vi "test_Loopback(Tx Generic - Rx Mon).vi"() -> ()   [LabVIEW 2020]
doc: "Overview: This examples helps to setup the board (or boards) and validate that it can send and receive parameters.\n\nRequirement: One AIM ARINC-664 board with installed AIM ARINC 664 BSP.\nRestrictions: None.\nInstruction:\n1. Select the Board ID (0 if you have only one board in your system) and the port number. If you want to validate between two ports in one device, you can use tx board and Rx Boardd\n2. Run the VI.\n3. See the result in the indicators.\nFor detailed information about functions use, see documents in <BSP Installation folder>\\AIM GmbH\\Arinc 664 Windows BSP <version>\\Doc."
uses:
  <instrlib>/AIM GmbH/_AIM 664/_controls/session_monitor_config.ctl
  <instrlib>/AIM GmbH/_AIM 664/_controls/queue_header_generic.ctl
  <instrlib>/AIM GmbH/_AIM 664/_controls/queue_data_full.ctl
  <instrlib>/AIM GmbH/_AIM 664/_controls/port_speed.ctl
  <instrlib>/AIM GmbH/_AIM 664/bsp/Fdx Create Session (RX-Monitor).vi
  <instrlib>/AIM GmbH/_AIM 664/bsp/Fdx Create Session (Tx-Generic).vi
  <instrlib>/AIM GmbH/_AIM 664/bsp/Fdx Start (Rx).vi
  <instrlib>/AIM GmbH/_AIM 664/bsp/Fdx Start (Tx).vi
  <instrlib>/AIM GmbH/_AIM 664/bsp/Fdx Stop (Tx).vi
  <instrlib>/AIM GmbH/_AIM 664/bsp/Fdx Stop (Rx).vi
  <instrlib>/AIM GmbH/_AIM 664/AIM664LV.lvlib
panel:
  in  "UDPsrcPort":u16=1
  in  "UDPdstPort":u16=1
  in  "Fdx configuration":T1={"domainID"=1, "sideID"=1, "locationID"=1, "interfaceID"=1, "partitionID"=1} {"interfaceID" format="%.0b"}
  in  "VL Id":u16=60
  out "EntryRead":u32
  out "BytesRead":u32
  out "Synchronized":u32
  out "ReadBuffer":u8[](array[numeric]) format="%.0x"
  out "Statistics":string[][](table)
  in  "MaxReadBytes":u32=257
  out "current time":timestamp
  out "tx timed out":bool
  out "rx timed out":bool
  in  "Data Payload":u8[](array[numeric])=[65, 66, 67, 68, 69, 70, 71, 72, 73, 74, 75, 76, 77, 78, 79, 80, 81] format="%.0x"
  in  "HeaderInfo":T2={"InterFrameGap"=1000, "PacketGroupWaitTime"=10000, "PayloadBufferMode"=0, "PayloadGenerationMode"=0, "PreambleCount"=0, "Skew"=1, "NetSelect"=0, "FrameStartMode"=1, "PhysErrorInjection"=0, "SequenceNumberInit"=65535, "SequenceNumberOffset"=65535} {"NetSelect" items=["FDX_TX_FRAME_DLY_A"=0, "FDX_TX_FRAME_DLY_B"=1, "FDX_TX_FRAME_BOTH "=3, "FDX_TX_FRAME_ONLY_A"=4, "FDX_TX_FRAME_ONLY_B "=5]; "FrameStartMode" items=["FDX_TX_FRAME_START_IFG", "FDX_TX_FRAME_START_PGWT", "FDX_TX_FRAME_START_TRG"]; "PhysErrorInjection" items=["FDX_TX_FRAME_ERR_OFF"=0, "FDX_TX_FRAME_ERR_CRC"=1, "FDX_TX_FRAME_ERR_ALI"=2, "FDX_TX_FRAME_ERR_PRE"=4, "FDX_TX_FRAME_ERR_PHY"=8]; "SequenceNumberInit" items=["FDX_TX_FRAME_SEQ_INIT_AUTO"=65535]; "SequenceNumberOffset" items=["FDX_TX_FRAME_SEQ_OFFS_AUTO "=65535]; "PayloadGenerationMode" items=["FDX_TX_FRAME_PGM_USER"=0, "FDX_TX_FRAME_PGM_IP_PART"=1, "FDX_TX_FRAME_PGM_IP_FULL"=2, "FDX_TX_FRAME_PGM_IP_PART_TT"=10, "FDX_TX_FRAME_PGM_IP_FULL_TT"=20]; "PayloadBufferMode" items=["FDX_TX_FRAME_PBM_STD", "FDX_TX_FRAME_PBM_MAC", "FDX_TX_FRAME_PBM_UDP"]}
  out "error out":errorcluster
  in  "EntryCount (1)":u32=1
  out "MonStatus":T3 {"MonStatus" items=["FDX_MON_OFF", "FDX_MON_WAIT_FOR_TRIGGER", "FDX_MON_TRIGGERED", "FDX_MON_STOPPED", "FDX_MON_FULL", "FDX_MON_OVERLOAD"]}
  in  "Control":u32(ring)=1 items=["FDX_RX_GS_RES_NO_CNT", "FDX_RX_GS_RES_ALL_CNT", "FDX_RX_GS_RES_ERR_CNT"]
  out "TxStatus":T4 {"TransmitMode" items=["FDX_TX_GENERIC", "FDX_TX_REPLAY", "FDX_TX_INDIVIDUAL"]; "TxStatus" items=["FDX_STAT_STOP", "FDX_STAT_RUN", "FDX_STAT_ERROR", "FDX_STAT_WAIT_F_TRIG"]}
  out "rx link ok":bool
  out "tx link ok":bool
  out "GlobMonSize":u32
  in  "RecordingFileName":path
  in  "MaxFileSize MB (1)":u32=1
  in  "Strobe":u32(ring) items=["FDX_MON_STROBE_DIS", "FDX_MON_STROBE_STOP", "FDX_MON_STROBE_START"]
  in  "CaptureMode":u32(ring) items=["FDX_MON_SINGLE ", "FDX_MON_CONTINUOUS", "FDX_MON_SELECTIVE", "FDX_MON_RECORDING", "FDX_MON_REROS", "FDX_MON_HMU"]
  in  "TriggerPosition":u32
  in  "MonitorConfig":T5={"DefaultCronoMode"=1, "GlbMonBufferSizeIn"=0} {"DefaultCronoMode" items=["FDX_RX_DEFAULT_ENA_CNT", "FDX_RX_DEFAULT_MON_ENA_ALL", "FDX_RX_DEFAULT_MON_ENA_GOOD"]}
  in  "Rx Port":u32=1
  in  "Rx Board":u32
  out "PortInitOut":T6 {"PortConfig" items=["FDX_SINGLE", "FDX_REDUNDANT"]}
  out "TxQueueInfo":cluster{"QueueBaseAddr":u32, "QueueSizeOut":u32}
  in  "Tx Board":u32
  in  "QueueSizeIn":u32
  in  "Tx Port":u32
  # "ARINC 664 Loopback"
  # "Overview: This examples helps to setup the board (or boards) and validate that it can send and receive parameters.\n\nRequirement: One AIM ARINC-664 board with installed AIM ARINC 664 BSP.\nRestrictions: None.\nInstruction:\n1. Select the Board ID (0 if you have only one board in your system) and the port number. If you want to validate between two ports in one device, you can use tx board and Rx Boardd\n2. Run the VI.\n3. See the result in the indicators."
  # "TX Status"
  # "Monitor Results"
  # "HW config"
  # "TX Configuration"
  # "Monitor Configuration"
  # "Monitor Status"
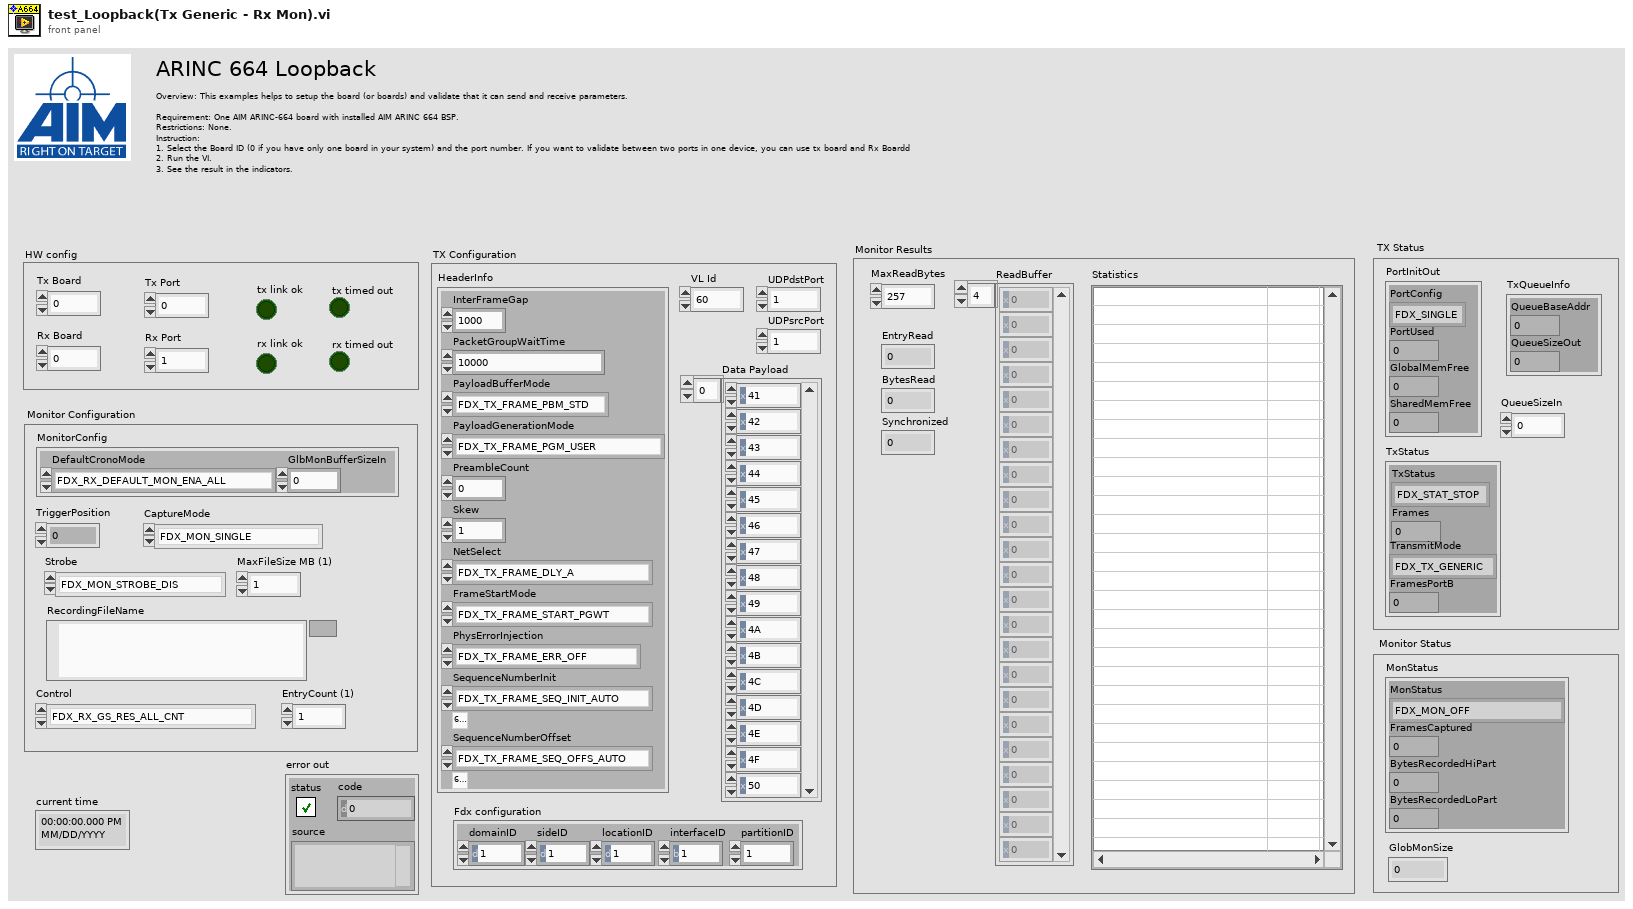
[diagram p1: front panel]
types:
  T1 = typedef "AIM664LV.lvlib/queue_data_full.ctl" = cluster{"domainID":u8, "sideID":u8, "locationID":u8, "interfaceID":u8, "partitionID":u8}
  T2 = typedef "AIM664LV.lvlib/queue_header_generic.ctl" = cluster{"InterFrameGap":u32, "PacketGroupWaitTime":u32, "PayloadBufferMode":u8, "PayloadGenerationMode":u8, "PreambleCount":u8, "Skew":u32, "NetSelect":u8, "FrameStartMode":u8, "PhysErrorInjection":u32, "SequenceNumberInit":u16, "SequenceNumberOffset":u16}
  T3 = cluster{"MonStatus":u32, "FramesCaptured":u32, "BytesRecordedHiPart":u32, "BytesRecordedLoPart":u32}
  T4 = cluster{"TxStatus":u32, "Frames":u32, "TransmitMode":u32, "FramesPortB":u32}
  T5 = typedef "AIM664LV.lvlib/session_monitor_config.ctl" = cluster{"DefaultCronoMode":u32, "GlbMonBufferSizeIn":u32}
  T6 = cluster{"PortConfig":u32, "PortUsed":u32, "GlobalMemFree":u32, "SharedMemFree":u32}
  T7 = typedef "AIM664LV.lvlib/port_speed.ctl" = u32
  T8 = cluster{"PortSpeed[0]":T7, "PortSpeed[1]":T7, "PortSpeed[2]":T7, "PortSpeed[3]":T7}
  T9 = cluster{"TotalByteCount":u32[], "FrameGoodCount":u32[], "FrameErrorCount":u32[], "BytesPerSecond":u32[], "FramesPerSecond":u32[], "PhysErrorCount":u32[], "PreamErrorCount":u32[], "UnaligErrorCount":u32[], "CRCErrorCount":u32[], "IFGErrorCount":u32[], "IPErrorCount":u32[], "MACErrorCount":u32[], "NoSfdErrorCount":u32[], "VLLenErrorCount":u32[], "SNIntegrityErrorCount":u32[], "TrafShapingViolationCount":u32[], "MAC1Short":u32[], "MAC64To127Count":u32[], "MAC128To255Count":u32[], "MAC256To511Count":u32[], "MAC512To1023Count":u32[], "MAC1024To1518Count":u32[], "MACLong":u32[]}
  T10 = cluster{"EntryRead":u32, "BytesRead":u32, "Synchronized":u32, "ReadBuffer":u8[]}
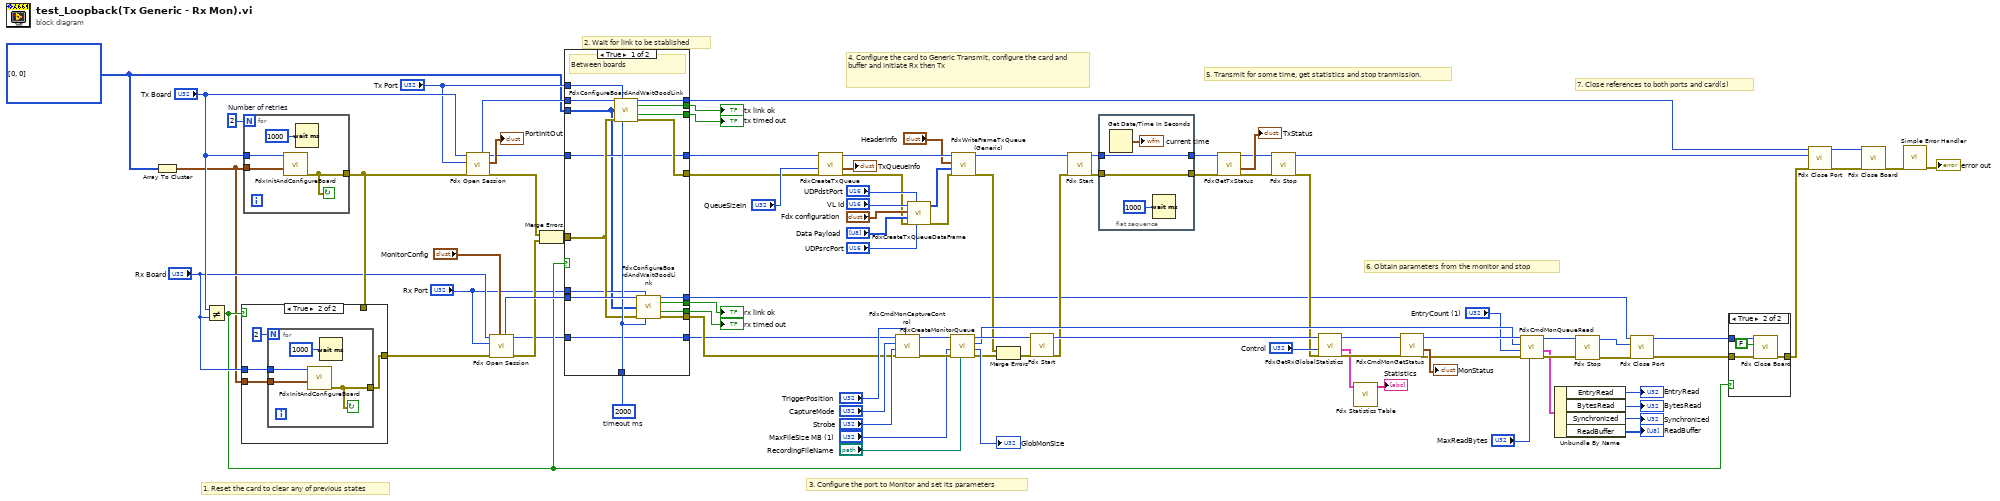
[diagram p0: block diagram]
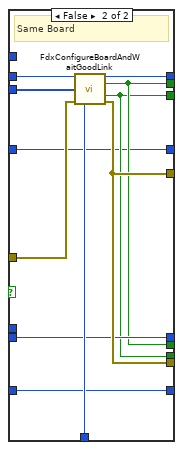
[diagram p3: hidden frame]
diagram:
  w4 = T7[] [0, 0] items=["FDX_100MBIT"=0, "FDX_10MBIT"=1, "FDX_1000MBIT"=5, "FDX_AUTO_100MBIT"=2, "FDX_AUTO_10MBIT"=3] ("PortSpeed")
  w34 = 2  # Number of retries
  w23 = u32 2000  # timeout ms
  # "7. Close references to both ports and card(s)"
  # "6. Obtain parameters from the monitor and stop"
  # "5. Transmit for some time, get statistics and stop tranmission."
  # "2. Wait for link to be stablished"
  # "3. Configure the port to Monitor and set its parameters"
  # "4. Configure the card to Generic Transmit, configure the card and buffer and initiate Rx then Tx"
  # "1. Reset the card to clear any of previous states"
  n1 = Array To Cluster(array=w4) -> (cluster=w3:T8)
  n2 = Not Equal?(x="Tx Board", y="Rx Board") -> (x != y?=w12:bool)
  n3 = for {
    N: w34 -> [_]
    tunnel: [w96] -> w32
    tunnel: "Tx Board" -> [w95]
    tunnel: w3 -> [w94]
    stop <- w96 continue-if-true
    n4 = call <instrlib>:"FdxInitAndConfigureBoard.vi"("PortSpeed (100Mbit)"=w94, "board index"=w95) -> ("error out"=w96:errorcluster)  [unwired: 5 in, 4 out]
    n5 = Wait (ms)(milliseconds to wait=u32 1000) -> ()  [unwired: 1 out]
  }
  n6 = case shown="True" w12 {
    tunnel: w32 -> [w98 _]
    tunnel: [w98 w100] -> w31
    tunnel: "Rx Board" -> [_ w101]
    tunnel: w3 -> [_ w99]
    frame False {
    }
    frame True {
      n7 = for {
        N: 2 -> [_]
        tunnel: [w105] -> w100
        tunnel: w101 -> [w104]
        tunnel: w99 -> [w103]
        stop <- w105 continue-if-true
        n8 = call <instrlib>:"FdxInitAndConfigureBoard.vi"("PortSpeed (100Mbit)"=w103, "board index"=w104) -> ("error out"=w105:errorcluster)  [unwired: 5 in, 4 out]
        n9 = Wait (ms)(milliseconds to wait=u32 1000) -> ()  [unwired: 1 out]
      }
    }
  }
  n10 = call-poly <instrlib>:"Fdx Open Session.vi"("error in (no error)"=w32, "port"="Tx Port", "board"="Tx Board") -> ("error out"=w22:errorcluster, "PortInitOut"=→"PortInitOut":T6, "port handle out"=w11:u32, "InstrumentHandle_board out"=w93:u32)  [unwired: 3 in, 2 out]
  n11 = call-poly <instrlib>:"Fdx Open Session.vi"("MonitorConfig"="MonitorConfig", "error in (no error)"=w31, "port"="Rx Port", "board"="Rx Board") -> ("error out"=w19:errorcluster, "InstrumentHandle_port out"=w9:u32, "InstrumentHandle_board out"=w80:u32)  [unwired: 2 in, 3 out]
  n12 = Merge Errors(w22, w19) -> (w18:errorcluster)
  n13 = case shown="True" w12 {
    tunnel: w93 -> [w123 w134]
    tunnel: w80 -> [w122 w129]
    tunnel: [w121 w128] -> w79
    tunnel: [w120 w133] -> w57
    tunnel: [w119 w129] -> w13
    tunnel: [w118 w127] -> w53
    tunnel: w23 -> [w117 w132]
    tunnel: [w116 w130] -> w21
    tunnel: [w115 w130] -> w20
    tunnel: w18 -> [w114 w131]
    tunnel: [w113 w128] -> w17
    tunnel: [w112 w127] -> w16
    tunnel: w11 -> [w111 w126]
    tunnel: [w111 w126] -> w10
    tunnel: w9 -> [w110 w125]
    tunnel: [w110 w125] -> w8
    tunnel: "Tx Port" -> [w109 _]
    tunnel: "Rx Port" -> [w108 _]
    tunnel: w4 -> [w107 w124]
    frame True {
      # "Between boards"
      n14 = call <instrlib>:"FdxConfigureBoardAndWaitGoodLink.vi"("InstrumentHandle_board in"=w123, "Port for Goodlink (-1 is all)"=w109, "PortSpeed"=w107, "error in"=w114, "timeout (ms)"=w117) -> ("InstrumentHandle_board out"=w120:u32, "good link"=w113:bool, "timed out"=w112:bool, "error out"=w116:errorcluster)  [unwired: 7 in]
      n15 = call <instrlib>:"FdxConfigureBoardAndWaitGoodLink.vi"("InstrumentHandle_board in"=w122, "Port for Goodlink (-1 is all)"=w108, "PortSpeed"=w107, "error in"=w114, "timeout (ms)"=w117) -> ("InstrumentHandle_board out"=w119:u32, "good link"=w121:bool, "timed out"=w118:bool, "error out"=w115:errorcluster)  [unwired: 7 in]
    }
    frame False {
      # "Same Board"
      n16 = call <instrlib>:"FdxConfigureBoardAndWaitGoodLink.vi"("InstrumentHandle_board in"=w134, "PortSpeed"=w124, "error in"=w131, "timeout (ms)"=w132) -> ("InstrumentHandle_board out"=w133:u32, "good link"=w128:bool, "timed out"=w127:bool, "error out"=w130:errorcluster)  [unwired: 8 in]
    }
  }
  "tx link ok" <- w17
  "rx link ok" <- w79
  "rx timed out" <- w53
  "tx timed out" <- w16
  n17 = call <instrlib>:"FdxCreateTxQueue.vi"("error in"=w21, "QueueSizeIn"="QueueSizeIn", "InstrumentHandle_port"=w10) -> ("error out"=w29:errorcluster, "TxQueueInfo"=→"TxQueueInfo":cluster{"QueueBaseAddr":u32, "QueueSizeOut":u32}, "InstrumentHandle_port"=w56:u32)  [unwired: 6 in]
  n18 = call <instrlib>:"FdxCmdMonCaptureControl.vi"("TriggerPosition"="TriggerPosition", "error in"=w20, "Strobe"="Strobe", "CaptureMode"="CaptureMode", "InstrumentHandle_port in"=w8) -> ("error out"=w84:errorcluster, "InstrumentHandle_port out"=w85:u32)  [unwired: 5 in]
  n19 = call <instrlib>:"FdxCreateTxQueueDataFrame.vi"("UDPsrcPort"="UDPsrcPort", "UDPdstPort"="UDPdstPort", "error in"=w29, "Payload"="Data Payload", "afdx configuration"="Fdx configuration", "VL Id"="VL Id") -> ("error out"=w28:errorcluster, "Frame"=w40:u8[])  [unwired: 3 in, 1 out]
  n20 = call <instrlib>:"FdxCreateMonitorQueue.vi"("RecordingFileName"="RecordingFileName", "error in (no error)"=w84, "MaxFileSize MB (1)"="MaxFileSize MB (1)", "InstrumentHandle_port in"=w85) -> ("error out"=w26:errorcluster, "GlobMonSize"=→"GlobMonSize":u32, "QueueIdOut"=w64:u32, "InstrumentHandle_port out"=w78:u32)  [unwired: 4 in]
  n21 = call <instrlib>:"FdxWriteFrameTxQueue (Generic).vi"("error in (no error)"=w28, "Frame in"=w40, "HeaderInfo"="HeaderInfo", "InstrumentHandle_port in"=w56) -> ("error out"=w24:errorcluster, "InstrumentHandle_port out"=w55:u32)  [unwired: 6 in]
  n22 = Merge Errors(w24, w26) -> (w25:errorcluster)
  n23 = call-poly <instrlib>:"Fdx Start.vi"("error in"=w25, "InstrumentHandle_port in"=w78) -> ("error out"=w51:errorcluster, "InstrumentHandle_port out"=w71:u32)  [unwired: 8 in]
  n24 = call-poly <instrlib>:"Fdx Start.vi"("error in"=w51, "InstrumentHandle_port in"=w55) -> ("error out"=w52:errorcluster, "InstrumentHandle_port out"=w77:u32)  [unwired: 8 in]
  n25 = flat-sequence {
    tunnel: w52 -> [w137]
    tunnel: [w137] -> w74
    tunnel: [w136] -> w75
    tunnel: w77 -> [w136]
    frame #0 {
      n26 = Get Date/Time In Seconds() -> (seconds since 1Jan1904=→"current time":timestamp)
      n27 = Wait (ms)(milliseconds to wait=u32 1000) -> ()  [unwired: 1 out]
    }
  }
  n28 = call <instrlib>:"FdxGetTxStatus.vi"("error in"=w74, "InstrumentHandle_port"=w75) -> ("error out"=w72:errorcluster, "TxStatus"=→"TxStatus":T4, "InstrumentHandle_port"=w73:u32)  [unwired: 7 in]
  n29 = call-poly <instrlib>:"Fdx Stop.vi"("error in"=w72, "InstrumentHandle_port in"=w73) -> ("error out"=w15:errorcluster, "InstrumentHandle_port out"=w58:u32)  [unwired: 8 in]
  n30 = call <instrlib>:"FdxGetRxGlobalStatistics.vi"("error in"=w15, "Control"="Control", "InstrumentHandle_port in"=w71) -> ("error out"=w68:errorcluster, "GlobalStat Out"=w46:T9, "InstrumentHandle_port out"=w69:u32)  [unwired: 6 in]
  n31 = call <instrlib>:"Fdx Statistics Table.vi"("Global Statistics"=w46) -> ("Table Control"=→"Statistics":string[][])  [unwired: 10 in]
  n32 = call <instrlib>:"FdxCmdMonGetStatus.vi"("error in"=w68, "InstrumentHandle_port in"=w69) -> ("error out"=w65:errorcluster, "MonStatus"=→"MonStatus":T3, "InstrumentHandle_port out"=w66:u32)  [unwired: 7 in]
  n33 = call <instrlib>:"FdxCmdMonQueueRead.vi"("MaxReadBytes"="MaxReadBytes", "error in"=w65, "EntryCount"="EntryCount (1)", "QueueId"=w64, "InstrumentHandle_port"=w66) -> ("error out"=w61:errorcluster, "QueueReadOut"=w45:T10, "InstrumentHandle_port"=w62:u32)  [unwired: 3 in, 1 out]
  n34 = Unbundle By Name(w45) -> ("EntryRead"=→"EntryRead":u32, "BytesRead"=→"BytesRead":u32, "Synchronized"=→"Synchronized":u32, "ReadBuffer"=→"ReadBuffer":u8[])
  n35 = call-poly <instrlib>:"Fdx Stop.vi"("error in"=w61, "InstrumentHandle_port in"=w62) -> ("error out"=w59:errorcluster, "InstrumentHandle_port out"=w60:u32)  [unwired: 8 in]
  n36 = call <instrlib>:"Fdx Close Port.vi"("error in"=w59, "InstrumentHandle_port in"=w60, "InstrumentHandle_board in"=w13) -> ("error out"=w14:errorcluster, "InstrumentHandle_board out"=w7:u32)  [unwired: 7 in]
  n37 = case shown="True" w12 {
    tunnel: w14 -> [w139 w143]
    tunnel: [w139 w142] -> w2
    tunnel: w7 -> [_ w141]
    frame False {
    }
    frame True {
      n38 = call <instrlib>:"Fdx Close Board.vi"("error in"=w143, "Force Board Release (F)"=FALSE ("Close reference to library?"), "InstrumentHandle_board in"=w141) -> ("error out"=w142:errorcluster)  [unwired: 8 in]
    }
  }
  n39 = call <instrlib>:"Fdx Close Port.vi"("error in"=w2, "InstrumentHandle_port in"=w58, "InstrumentHandle_board in"=w57) -> ("error out"=w50:errorcluster, "InstrumentHandle_board out"=w27:u32)  [unwired: 7 in]
  n40 = call <instrlib>:"Fdx Close Board.vi"("error in"=w50, "InstrumentHandle_board in"=w27) -> ("error out"=w1:errorcluster)  [unwired: 9 in]
  n41 = call <vilib>:"Simple Error Handler.vi"("error in (no error)"=w1) -> ("error out"=→"error out":errorcluster)  [unwired: 4 in, 4 out]
